vi "9_nov_LOOP.vi"() -> ()   [LabVIEW 2020]
uses:
  <instrlib>/Agilent B2900 Series/Public/Configure/Measurement/Configure Measurement (Resistance).vi
  <instrlib>/Agilent B2900 Series/Public/Data/Read Measurement Result (Single Point).vi
  <instrlib>/Agilent B2900 Series/Agilent B2900 Series.lvlib
panel:
  in  "Channel (0: Channel 1)":i32(ring) items=["Channel 1", "Channel 2"]
  out "Voltage":dbl(graph)
  out "Current":dbl(graph)
  out "XY Graph":cluster{"X":dbl[], "Y":dbl[]}[](graph)
  in  "stop":bool
  out "Measured Current (A)":dbl
  out "Measured Voltage (Volts)":dbl
  in  "Enable Current Measurement (T: Enable)":bool=TRUE
  in  "Enable Voltage Measurement (T: Enable)":bool=TRUE
  in  "Enable Resistance Measurement (F: Disable)":bool
  in  "SELECT DEVICE":refnum<visa-resource-name>="COM1"
  out "Measured Resistance (ohms)":dbl
  # "Configuration"
  # "MEASURED VALUES"
  # "ENABLE MODES"
  # "Y"
  # "X"
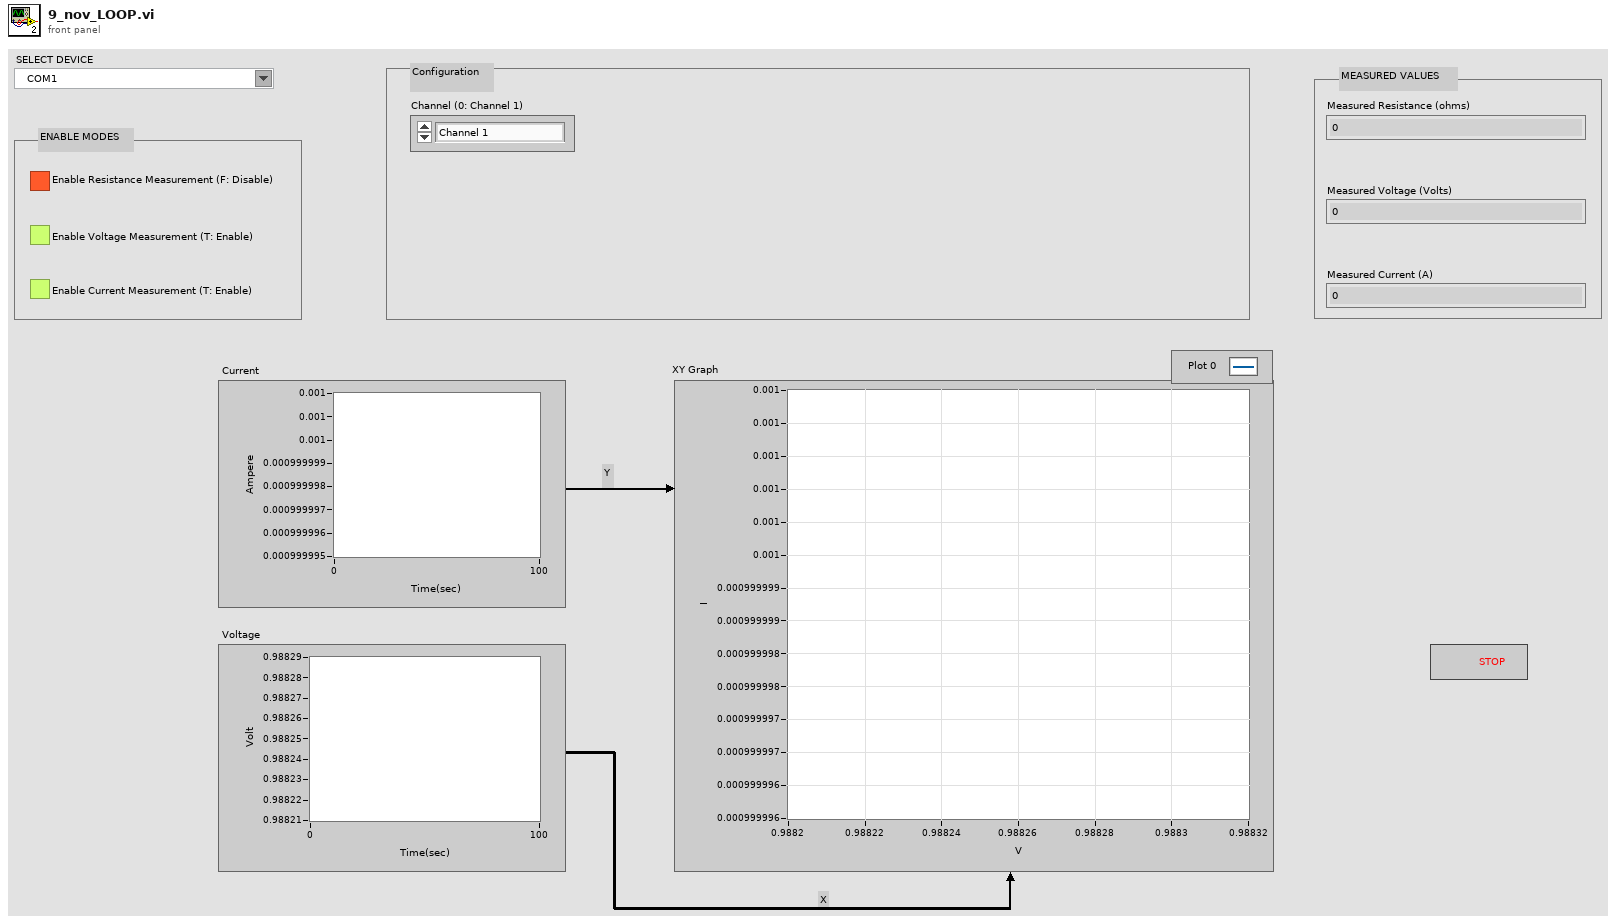
[diagram p1: front panel]
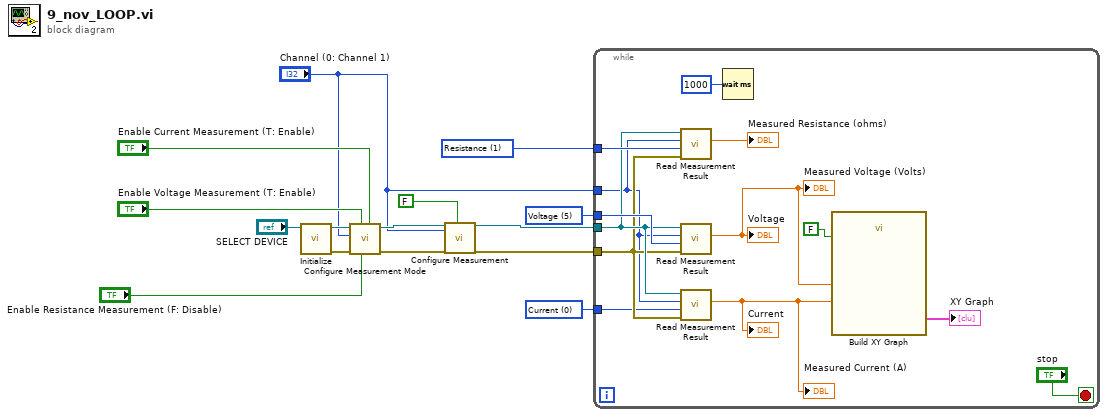
[diagram p0: block diagram]
diagram:
  w2 = 0 items=["Current", "Resistance", "Source Output Setting", "Status", "Time", "Voltage"] ("Data Mode (5: Voltage)")
  w5 = 5 items=["Current", "Resistance", "Source Output Setting", "Status", "Time", "Voltage"] ("Data Mode (5: Voltage)")
  w15 = 1 items=["Current", "Resistance", "Source Output Setting", "Status", "Time", "Voltage"] ("Data Mode (5: Voltage)")
  n1 = call <instrlib>:"Initialize.vi"("VISA resource name"="SELECT DEVICE") -> ("error out"=w6:errorcluster, "VISA resource name out"=w7:refnum<visa-resource-name>)  [unwired: 9 in]
  n2 = call <instrlib>:"Configure Measurement Mode.vi"("Enable Current Measurement (T: Enable)"="Enable Current Measurement (T: Enable)", "Enable Resistance Measurement (F: Disable)"="Enable Resistance Measurement (F: Disable)", "Enable Voltage Measurement (T: Enable)"="Enable Voltage Measurement (T: Enable)", "error in (no error)"=w6, "Channel (0: Channel 1)"="Channel (0: Channel 1)", "VISA resource name"=w7) -> ("error out"=w13:errorcluster, "VISA resource name out"=w14:refnum<visa-resource-name>)  [unwired: 4 in]
  n3 = call-poly <instrlib>:"Configure Measurement.vi"("VISA resource name"=w14, "Channel (0: Channel 1)"="Channel (0: Channel 1)", "error in (no error)"=w13, "Enable Resistance Compensation (F: Disable)"=FALSE) -> ("VISA resource name out"=w4:refnum<visa-resource-name>, "error out"=w3:errorcluster)  [unwired: 14 in]
  n4 = while {
    tunnel: w15 -> [w28]
    tunnel: w5 -> [w27]
    tunnel: w4 -> [w26]
    tunnel: w3 -> [w25]
    tunnel: w2 -> [w24]
    tunnel: "Channel (0: Channel 1)" -> [w23]
    stop <- "stop" stop-if-true
    n5 = call-poly <instrlib>:"Read Measurement Result.vi"("error in (no error)"=w25, "Data Mode (5: Voltage)"=w28, "Channel (0: Channel 1)"=w23, "VISA resource name"=w26) -> ("Measurement Result"=→"Measured Resistance (ohms)":dbl)  [unwired: 5 in, 2 out]
    n6 = call-poly <instrlib>:"Read Measurement Result.vi"("error in (no error)"=w25, "Data Mode (5: Voltage)"=w27, "Channel (0: Channel 1)"=w23, "VISA resource name"=w26) -> ("Measurement Result"=w16:dbl)  [unwired: 5 in, 2 out]
    "Measured Voltage (Volts)" <- w16
    "Voltage" <- w16
    n7 = call-poly <instrlib>:"Read Measurement Result.vi"("error in (no error)"=w25, "Data Mode (5: Voltage)"=w24, "Channel (0: Channel 1)"=w23, "VISA resource name"=w26) -> ("Measurement Result"=w17:dbl)  [unwired: 5 in, 2 out]
    "Measured Current (A)" <- w17
    "Current" <- w17
    n8 = Wait (ms)(milliseconds to wait=u32 1000) -> ()  [unwired: 1 out]
    n9 = call "Build XY Graph"("Reset"=FALSE, "Y Input"=w17, "X Input"=w16) -> ("XY Graph"=→"XY Graph":cluster{"X":dbl[], "Y":dbl[]}[])  [unwired: 7 in, 1 out]
  }
